vi "dot_product_packet_nuevo.vi"(0 "x":u32, 1 "y":u32, 2 "width":u16) -> (8 "out":u64, 9 "valid":bool)   [LabVIEW 2017]
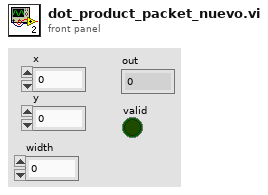
[diagram p1: front panel]
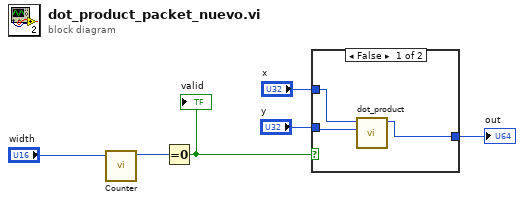
[diagram p0: block diagram]
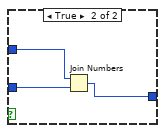
[diagram p2: hidden frame]
diagram:
  n1 = call "Counter.vi"("limit"="width") -> ("count"=w6:u16)  [unwired: 10 in]
  n2 = Equal To 0?(x=w6) -> (x = 0?=w4:bool)
  "valid" <- w4
  n3 = case shown="False" w4 {
    tunnel: [w9 w10] -> w3
    tunnel: "x" -> [w8 w12]
    tunnel: "y" -> [w7 w11]
    frame False {
      n4 = call "dot_product.vi"("y"=w7, "x"=w8) -> ("out"=w9:u64)  [unwired: 9 in]
    }
    frame True {
      n5 = Join Numbers(hi=w12, lo=w11) -> ((hi.lo)=w10:u64)
    }
  }
  "out" <- w3
